vi "rs3 get frame timestamp3.vi"(8 "error in (no error)":errorcluster, 11 "frame in":u64) -> (0 "error out":errorcluster, 1 "error":u64, 2 "Time stamp":dbl, 3 "frame out":u64)   [LabVIEW 2023]
doc: "Provides timestamp"
panel:
  # "RS3 Get Frame Timestamp 2"
  # "(C) Intel Corp.,  AGJ"
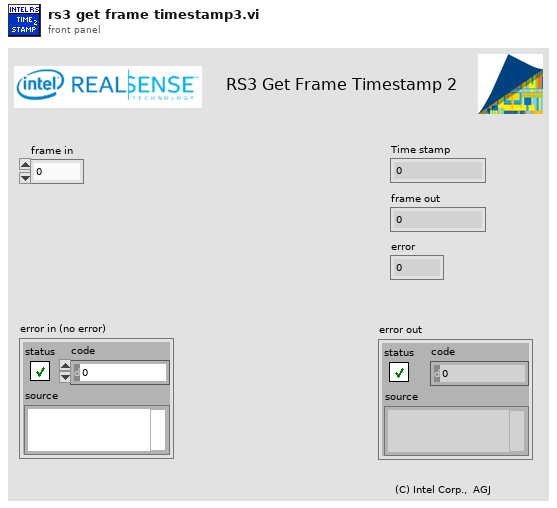
[diagram p1: front panel]
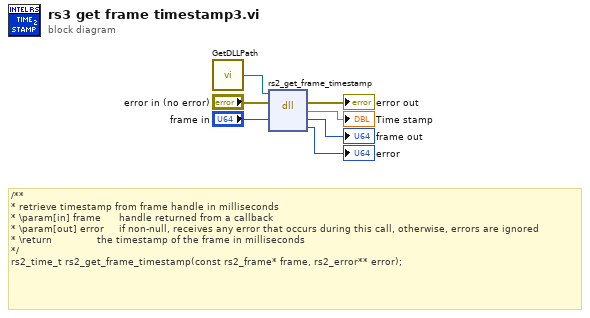
[diagram p0: block diagram]
diagram:
  # "/**\n* retrieve timestamp from frame handle in milliseconds\n* \\param[in] frame      handle returned from a callback\n* \\param[out] error     if non-null, receives any error that occurs during this call, otherwise, errors are ignored\n* \\return               the timestamp of the frame in milliseconds\n*/\nrs2_time_t rs2_get_frame_timestamp(const rs2_frame* frame, rs2_error** error);"
  n1 = call "GetDLLPath.vi"() -> ("DLL Path"=w1:path)
  n2 = dll-call lib="C:/STEAMSyndicate/RealSenseWrappers/VI Wrappers (add ons) Public/RealSense/realsense2.dll" fn="rs2_get_frame_timestamp"(path in=w1, error in="error in (no error)", "frame"="frame in") -> (error out=→"error out":errorcluster, "timestamp ms"=→"Time stamp":dbl, "frame"=→"frame out":u64, "error"=→"error":u64)  [unwired: 2 in, 1 out]
